vi "Test Count Number of Tests Enumerated.vi"(8 "error in (no error)":errorcluster, 11 "Result Model Tests in":refnum<class "Result Model Statistics.lvclass">) -> (0 "error out":errorcluster, 3 "Result Model Tests out":refnum<class "Result Model Statistics.lvclass">)   [LabVIEW 2020, in "Result Model Statistics.lvclass"]
uses:
  Result Model Statistics.lvclass
  206db1ee-aa99-40b9-8881-171f2a77c34b.vi
  source/User Interface/Result Model/Result Model.lvclass
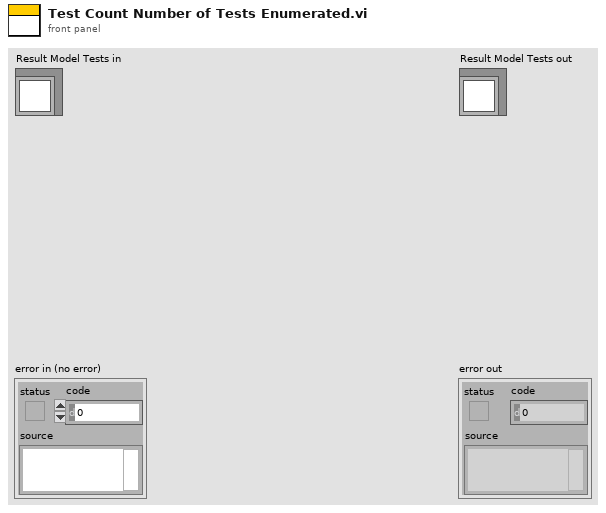
[diagram p1: front panel]
types:
  T1 = typedef "Result Model.lvclass/Statistics.ctl" = cluster{"Method Count":u32, "Executed Methods":u32, "Passed Methods":u32, "Failed Methods":u32, "Method Errors":u32, "Skipped Method":u32, "Progress [%]":dbl}
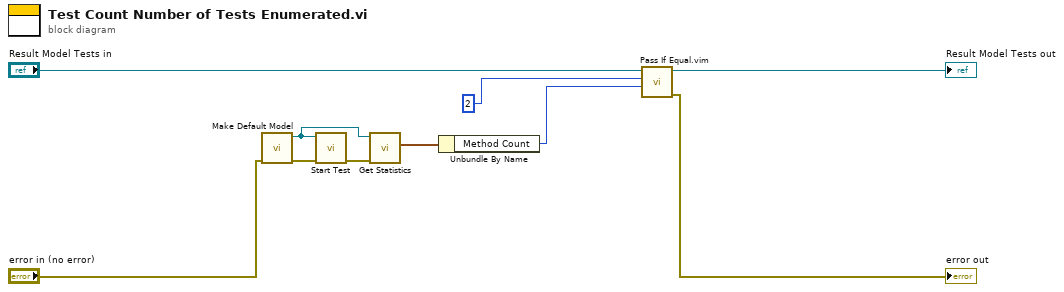
[diagram p0: block diagram]
diagram:
  n1 = call "Make Default Model.vi"("error in (no error)"="error in (no error)") -> ("error out"=w3:errorcluster, "Result Model out"=w1:refnum<class "Result Model.lvclass">)  [unwired: 9 in]
  n2 = call "Start Test.vi"("error in (no error)"=w3, "Result Model by Reference In"=w1) -> ("error out"=w2:errorcluster)  [unwired: 9 in]
  n3 = call "Get Statistics.vi"("error in (no error)"=w2, "Result Model in"=w1) -> ("Results"=w6:T1)  [unwired: 8 in, 1 out]
  n4 = Unbundle By Name(w6) -> ("Method Count"=w5:u32)
  n5 = call "Pass If Equal.vim"("Actual"=w5, "Expected"=u32 2 ("Method Count"), "LUnit Test Case In"="Result Model Tests in") -> ("error out"=→"error out":errorcluster, "LUnit Test Case Out"=→"Result Model Tests out":refnum<class "Result Model Statistics.lvclass">)  [unwired: 7 in]
